vi "S2C_M2p5942_Proc_Measure.vi"(7 "Command":string, 8 "Error In":errorcluster, 10 "Force Trigger?":bool, 11 "Card In":cluster{"Card Handle":u64, "Error Code":u32}) -> (0 "Error Out":errorcluster, 2 "Ready?":bool, 3 "Card Out":cluster{"Card Handle":u64, "Error Code":u32})   [LabVIEW 2024]
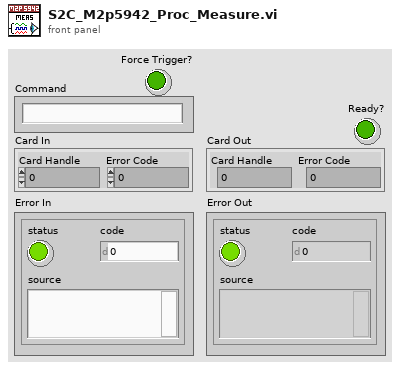
[diagram p1: front panel]
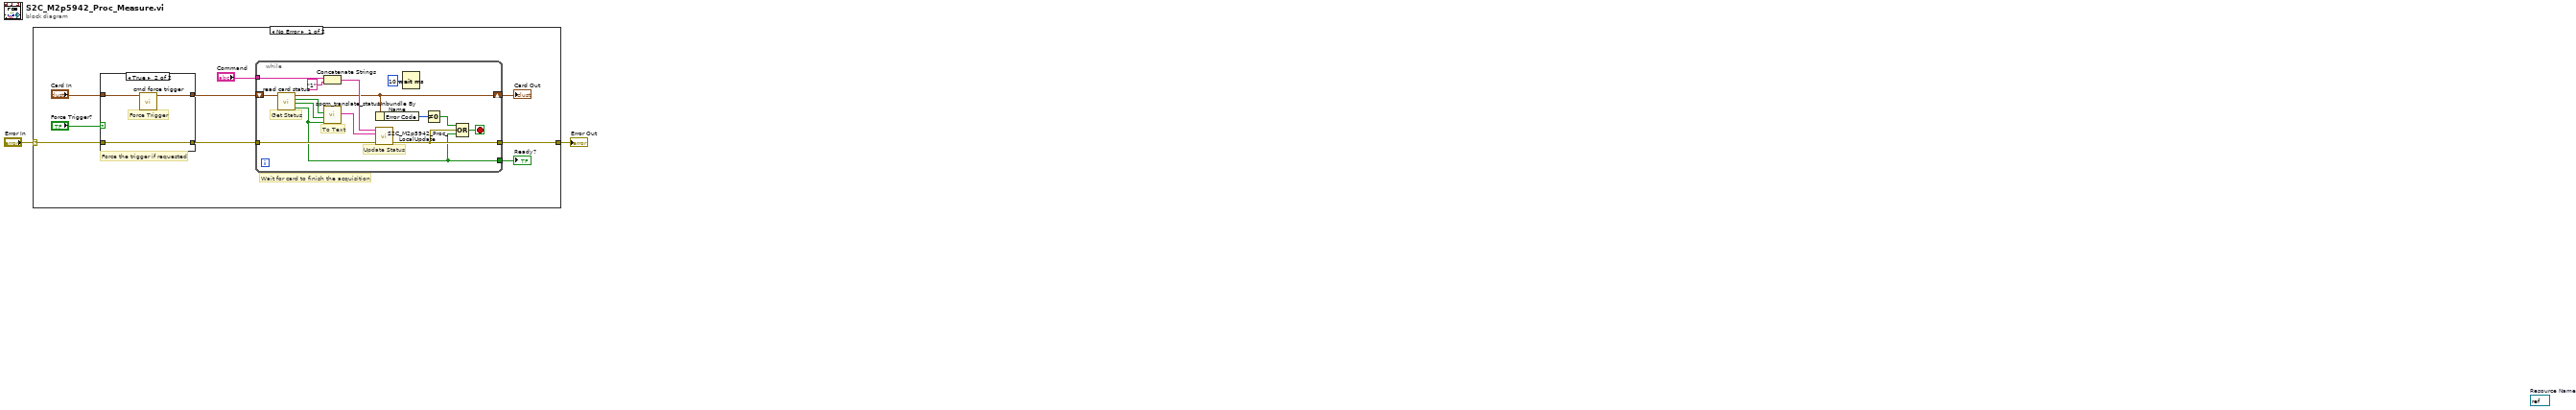
[diagram p0: block diagram]
diagram:
  (unwired) refnum<visa-resource-name> refnum  # Resource Name
  n1 = case shown="No Error" "Error In" {
    selector: "Error In" -> [w8 w32]
    tunnel: [w9 w32] -> w1
    frame No Error {
      # "Force the trigger if requested"
      # "Wait for card to finish the acquisition"
      n2 = case shown="True" "Force Trigger?" {
        tunnel: [w12 w16] -> w10
        tunnel: w8 -> [w13 w14]
        tunnel: [w13 w14] -> w6
        tunnel: "Card In" -> [w12 w15]
        frame False {
        }
        frame True {
          # "Force Trigger"
          n3 = call "cmd force trigger.vi"("Card Info In"=w15) -> ("Card Info Out"=w16:cluster{"Card Handle":u64, "Error Code":u32})  [unwired: 6 in]
        }
      }
      n4 = while {
        tunnel: "Command" -> [w23]
        tunnel: [w27] -> w9
        shift-right: [w19] -> w3
        shift-left: w10 -> [w29]
        tunnel: w6 -> [w20]
        tunnel: [w17] -> w5
        stop <- w26 stop-if-true
        # "Update Status"
        # "To Text"
        # "Get Status"
        n5 = call "read card status.vi"("Card Info In"=w29) -> ("Card ready"=w17:bool, "Trigger detected"=w31:bool, "Pretrigger full"=w30:bool, "Card Info Out"=w19:cluster{"Card Handle":u64, "Error Code":u32})  [unwired: 3 in]
        n6 = Concatenate Strings(w23, "1" ("string")) -> (w22:string)
        n7 = call "spcm_translate_status.vi"("Ready"=w17, "Trigger"=w31, "Pretrigger"=w30) -> ("Text"=w28:string)  [unwired: 4 in]
        n8 = Unbundle By Name(w19) -> ("Error Code"=w18:u32)
        n9 = call "S2C_M2p5942_Proc_LocalUpdate.vi"("Error In"=w20, "Data"=w28, "Command"=w22) -> ("Error Out"=w27:errorcluster)  [unwired: 8 in]
        n10 = Wait (ms)(milliseconds to wait=u32 10) -> ()  [unwired: 1 out]
        n11 = Not Equal To 0?(x=w18) -> (x != 0?=w21:bool)
        n12 = Compound Arithmetic op=OR(w21, w27, w17) -> (w26:bool)
      }
      "Ready?" <- w5
      "Card Out" <- w3
    }
    frame Error {
    }
  }
  "Error Out" <- w1
